vi "%s (Request).vi"(8 "error in (no error)":errorcluster, 11 "API-Reference in":refnum<data-value>) -> (0 "error out":errorcluster, 3 "API-Reference out":refnum<data-value>)   [LabVIEW 2018, in "Scripting.lvlib" / "Actor.lvclass"]
uses:
  Actor.lvclass
  Request-Enqueuers.ctl
  Did Stop.ctl
  API-Data.ctl
  Front-Panel State.ctl
  Did Initialize.ctl
  Broadcast Enqueuers.ctl
  All-Enqueuers.ctl
  State.ctl
  Get State.ctl
  Stop.ctl
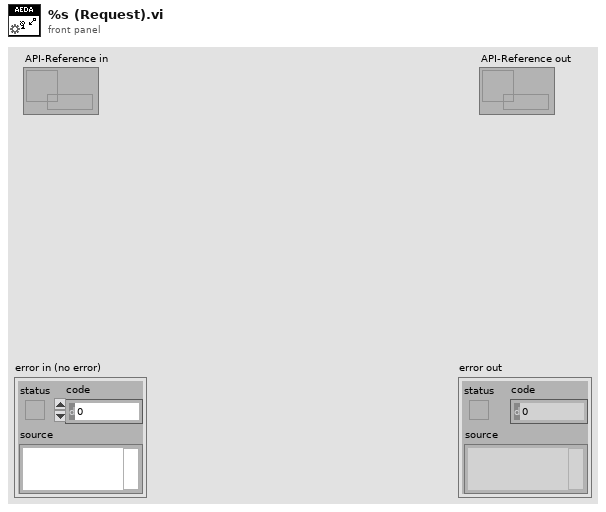
[diagram p1: front panel]
types:
  T1 = typedef "Scripting.lvlib/Actor.lvclass/API-Data.ctl" = cluster{"Launch":refnum<notifier>, "Did Stop Message":refnum<event-registration>, "Did Stop Enqueuer":refnum<user-event>, "Enqueuers":T2}
  T2 = typedef "Scripting.lvlib/Actor.lvclass/All-Enqueuers.ctl" = cluster{"Broadcasts":T3, "Requests":T4}
  T3 = typedef "Scripting.lvlib/Actor.lvclass/Broadcast Enqueuers.ctl" = cluster{"Did Initialize":refnum<user-event>}
  T4 = typedef "Scripting.lvlib/Actor.lvclass/Request-Enqueuers.ctl" = cluster{"Get State":refnum<user-event>, "Stop":refnum<user-event>}
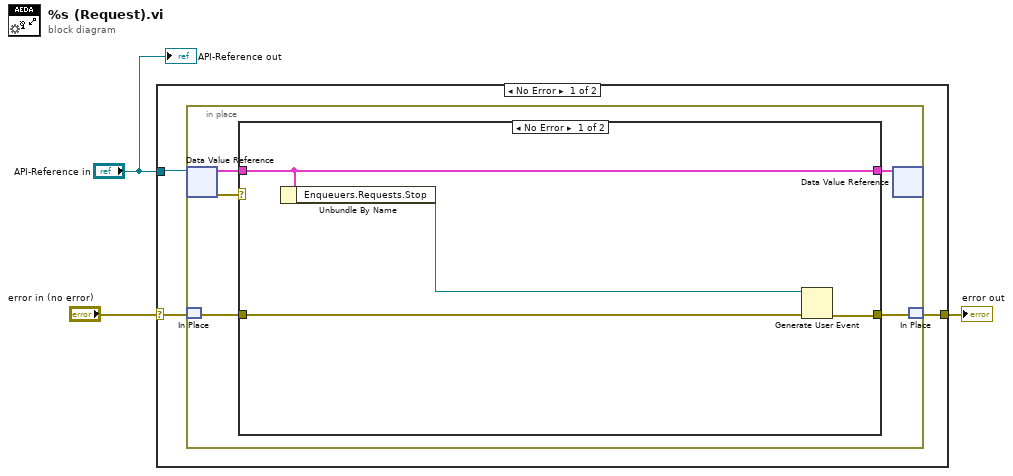
[diagram p0: block diagram]
diagram:
  n1 = case shown="No Error" "error in (no error)" {
    selector: "error in (no error)" -> [w6 w18]
    tunnel: [w5 w18] -> w2
    tunnel: "API-Reference in" -> [w4 _]
    frame No Error {
      n2 = in-place {
        n3 = in-place-dvr #1(w4) -> (w10:T1, w11:errorcluster)
        n4 = in-place-match #2(w6) -> (w8:errorcluster)
        n5 = case shown="No Error" w11 {
          selector: w11 -> [_ w17]
          tunnel: w10 -> [w15 w16]
          tunnel: [w15 w16] -> w9
          tunnel: w8 -> [w12 _]
          tunnel: [w14 w17] -> w7
          frame No Error {
            n6 = Unbundle By Name(w15) -> ("Enqueuers.Requests.Stop"=w13:refnum<user-event>)
            n7 = Generate User Event(user event=w13, error in=w12) -> (error out=w14:errorcluster)  [unwired: 2 in, 1 out]
          }
          frame Error {
          }
        }
        n8 = in-place-dvr #1(w9) -> ()  [unwired: 2 out]
        n9 = in-place-match #2(w7) -> (w5:errorcluster)
      }
    }
    frame Error {
    }
  }
  "error out" <- w2
  "API-Reference out" <- "API-Reference in"
